vi "Index Steps.vi"(8 "error in (no error)":errorcluster, 10 "Index":i32, 11 "Macro in":refnum<class "Macro.lvclass">) -> (0 "error out":errorcluster, 2 "Step":refnum<class "Step.lvclass">, 3 "Macro out":refnum<class "Macro.lvclass">)   [LabVIEW 2020, in "MacroAssert.lvlib" / "Macro.lvclass"]
doc: "Indexes the steps of <B>Macro in</B> at <B>Index</B>."
uses:
  Macro.lvclass
  Step/Step.lvclass
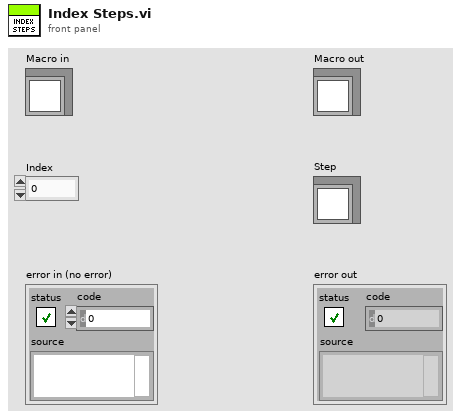
[diagram p1: front panel]
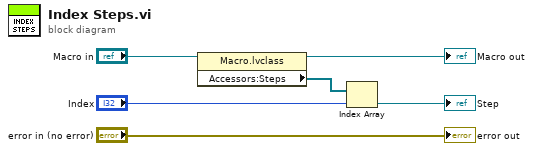
[diagram p0: block diagram]
diagram:
  n1 = property class="Macro.lvclass"(reference="Macro in") -> (reference out=→"Macro out":refnum<class "Macro.lvclass">, "Accessors:Steps"=w1:refnum<class "Step.lvclass">[])  [unwired: 1 in, 1 out]
  n2 = Index Array(array=w1, index="Index") -> (element=→"Step":refnum<class "Step.lvclass">)
  "error out" <- "error in (no error)"
